vi "Get DDS Modulus.vi"(8 "error in (no error)":errorcluster, 9 "Module":i32, 10 "Original DDS modulus":u32=1 format="0x%x (%d)", 11 "RP Instrument in":refnum<class "RP Instrument.lvclass">) -> (0 "error out":errorcluster, 2 "DDS modulus":i64, 3 "RP Instrument out":refnum<class "RP Instrument.lvclass">)   [LabVIEW 2024, in "RP Instrument.lvclass"]
uses:
  RP Instrument.lvclass
  RP Status Offsets.ctl
  RP Instrument.lvclass/RP Instrument.ctl
  <vilib>/ErrorRing/Error Ring.xnode
  RP Communicator/RP Communicator.lvclass
  <vilib>/Utility/error.llb/Error Cluster From Error Code.vi
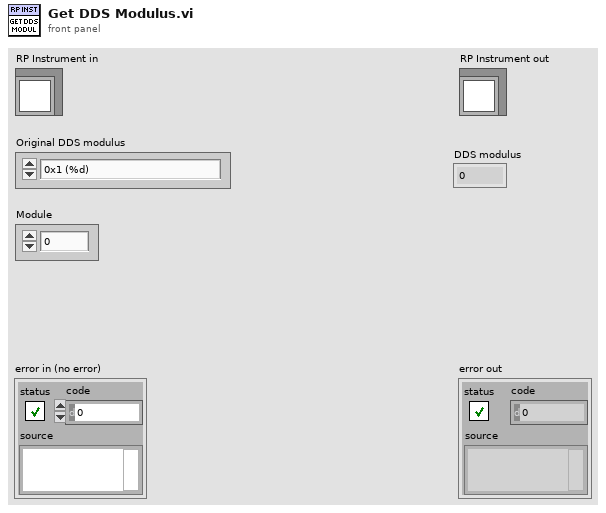
[diagram p1: front panel]
types:
  T1 = typedef "RP Status Offsets.ctl" = u16
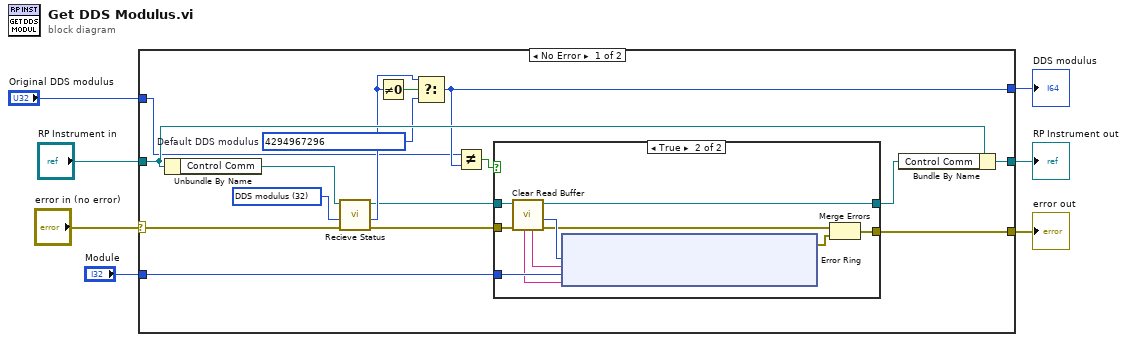
[diagram p0: block diagram]
diagram:
  n1 = case shown="No Error" "error in (no error)" {
    selector: "error in (no error)" -> [w19 w47]
    tunnel: [w11 w47] -> w6
    tunnel: [w20 w46] -> w4
    tunnel: "RP Instrument in" -> [w23 w46]
    tunnel: [w14 _] -> w3
    tunnel: "Original DDS modulus" -> [w13 _]
    tunnel: "Module" -> [w10 _]
    frame No Error {
      w16 = i64 4294967296  # Default DDS modulus
      w22 = T1 32 items=["Writer address"=0, "Record start position"=4, "Trig state and ID"=8, "Phase"=12, "X1"=16, "Y1"=20, "RxFIFO counter or  X2"=24, "TxFIFO counter or Y2"=28, "DDS modulus"=32] ("Status offsets")
      n2 = Unbundle By Name(w23) -> ("Control Comm"=w21:refnum<class "RP Communicator.lvclass">)
      n3 = call-dynamic "Recieve Status.vi"("error in (no error)"=w19, "Status offset"=w22, "RP Communicator in"=w21) -> ("error out"=w12:errorcluster, "Status response"=w17:u32, "RP Communicator out"=w9:refnum<class "RP Communicator.lvclass">)  [unwired: 6 in]
      n4 = Not Equal To 0?(x=w17) -> (x != 0?=w18:bool)
      n5 = Select(t=w17, s=w18, f=w16) -> (s? t:f=w14:i64)
      n6 = Not Equal?(x=w13, y=w14) -> (x != y?=w15:bool)
      n7 = case shown="True" w15 {
        tunnel: w12 -> [w25 w31]
        tunnel: [w25 w35] -> w11
        tunnel: w10 -> [_ w30]
        tunnel: w9 -> [w24 w33]
        tunnel: [w24 w32] -> w8
        frame False {
        }
        frame True {
          n8 = call-dynamic "Clear Read Buffer.vi"("error in (no error)"=w31, "RP Communicator in"=w33) -> ("error out"=w28:errorcluster, "bytes read"=w29:i32, "RP Communicator out"=w32:refnum<class "RP Communicator.lvclass">, "hex bytes"=w27:string, "Server address"=w26:string)  [unwired: 4 in, 1 out]
          n9 = xnode "Error Ring"("parameter 0"=w29, "parameter 1"=w27, "parameter 2"=w30, "parameter 3"=w26) -> ("error out"=w34:errorcluster)
          n10 = Merge Errors(w28, w34) -> (w35:errorcluster)
        }
      }
      n11 = Bundle By Name(cluster=w23, "Control Comm"=w8) -> (w20:refnum<class "RP Instrument.lvclass">)
    }
    frame Error {
    }
  }
  "error out" <- w6
  "RP Instrument out" <- w4
  "DDS modulus" <- w3
